vi "Start Module.vi"(6 "Show Main VI Diagram on Init (F)":bool, 8 "error in":errorcluster, 9 "Target UDP connection ref":refnum<k16>, 10 "IP:Port:Master/Slave":string, 11 "Run as Singleton? (F)":bool) -> (0 "error out":errorcluster, 1 "Wait for Event Sync?":bool, 2 "RT Interpreter Broadcast Events":T1, 3 "Module ID":i32, 4 "Module Name":string)   [LabVIEW 2021, in "RT Interpreter.lvlib"]
doc: "Launches an instance of the module Main VI. After calling this VI, you can optionally register for broadcast events from the module by wiring the broadcast events output of this VI to a <b>Register For Events</b> function. \n\nAfter the optional Register For Events function call, you should always call the <b>Synchronize Module Events.vi</b> for this module with the 'Wait for Event Sync?' output of this VI to the corresponding input of the Synchronize Module Events.vi. \n\nTo see an example of the proper wiring pattern, see the \"Run New Module: Value Change\" event frame in the API Tester VI for this module.\n\nThe <b>Validate DQMH Module</b> tool added a 'Module Name' output to this VI.\n_____\nBased on DQMH Dev Tools: Project Template 7.1.2.1547."
uses:
  RT Interpreter.lvlib
  Broadcast Events--cluster.ctl
  Did Init Argument--cluster.ctl
  Status Updated Argument--cluster.ctl
  Error Reported Argument--cluster.ctl
  Stop Argument--cluster.ctl
  Get Module Execution Status Argument--cluster.ctl
  Module Running State--enum.ctl
  <vilib>/Delacor/Delacor QMH/Libraries/Cloneable Module Admin_class/Delacor_lib_QMH_Cloneable Module Admin.lvclass
  C:/Program Files (x86)/National Instruments/LabVIEW 2021/vi.lib/Delacor/Delacor QMH/Libraries/Module Admin_class/Delacor_lib_QMH_Module Admin.lvclass
  VI Reference Management/Main VI Type--strict_vi_ref.ctl
  <vilib>/Delacor/Delacor QMH/Libraries/Cloneable Module Admin_class/Delacor_lib_QMH_Cloneable Module Admin.lvclass/Delacor_lib_QMH_Cloneable Module Admin.ctl
  <vilib>/Delacor/Delacor QMH/Libraries/Module Admin_class/Delacor_lib_QMH_Module Admin.lvclass/Delacor_lib_QMH_Module Admin.ctl
  <vilib>/Delacor/Delacor QMH/Libraries/Cloneable Module Admin_class/Delacor_lib_QMH_Set Module ID.vi
  <vilib>/Delacor/Delacor QMH/Libraries/Module Admin_class/Delacor_lib_QMH_Set External Launch.vi
  Main.vi
  Clone Registration/Clone Registration.lvlib
  VI Reference Management/VI Reference Management.lvlib
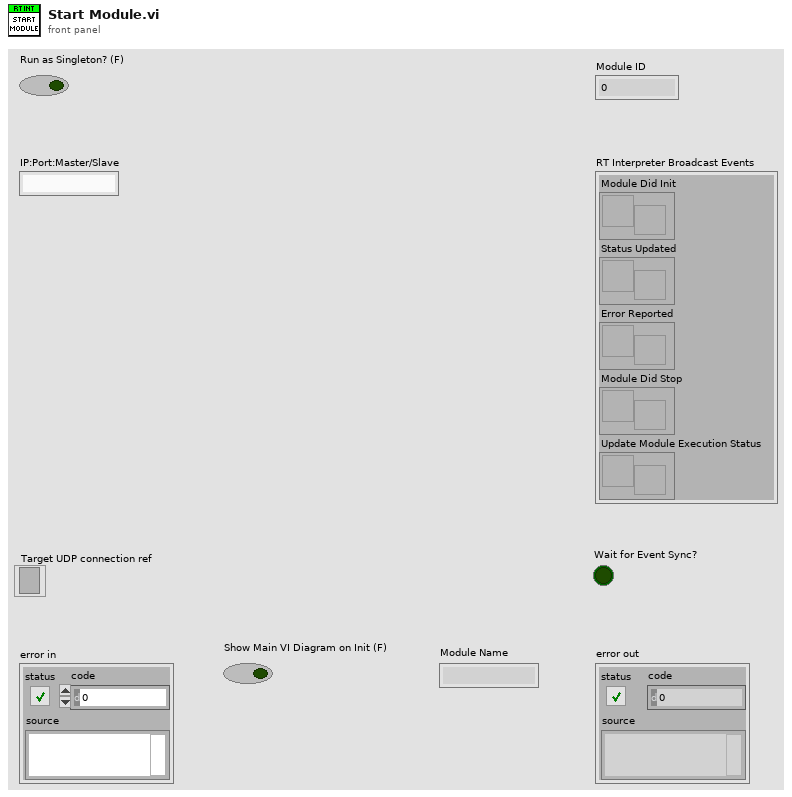
[diagram p1: front panel]
types:
  T1 = typedef "RT Interpreter.lvlib/Broadcast Events--cluster.ctl" = cluster{"Module Did Init":refnum<user-event>, "Status Updated":refnum<user-event>, "Error Reported":refnum<user-event>, "Module Did Stop":refnum<user-event>, "Update Module Execution Status":refnum<user-event>}
  T2 = typedef "RT Interpreter.lvlib/Module Running State--enum.ctl" = enum16{"Not Running", "Running as Cloneable", "Running as Singleton"}
  T3 = enum32{"Bad", "Idle", "Run top level", "Running"}
  T4 = typedef "RT Interpreter.lvlib/VI Reference Management.lvlib/Main VI Type--strict_vi_ref.ctl" = refnum<vi>
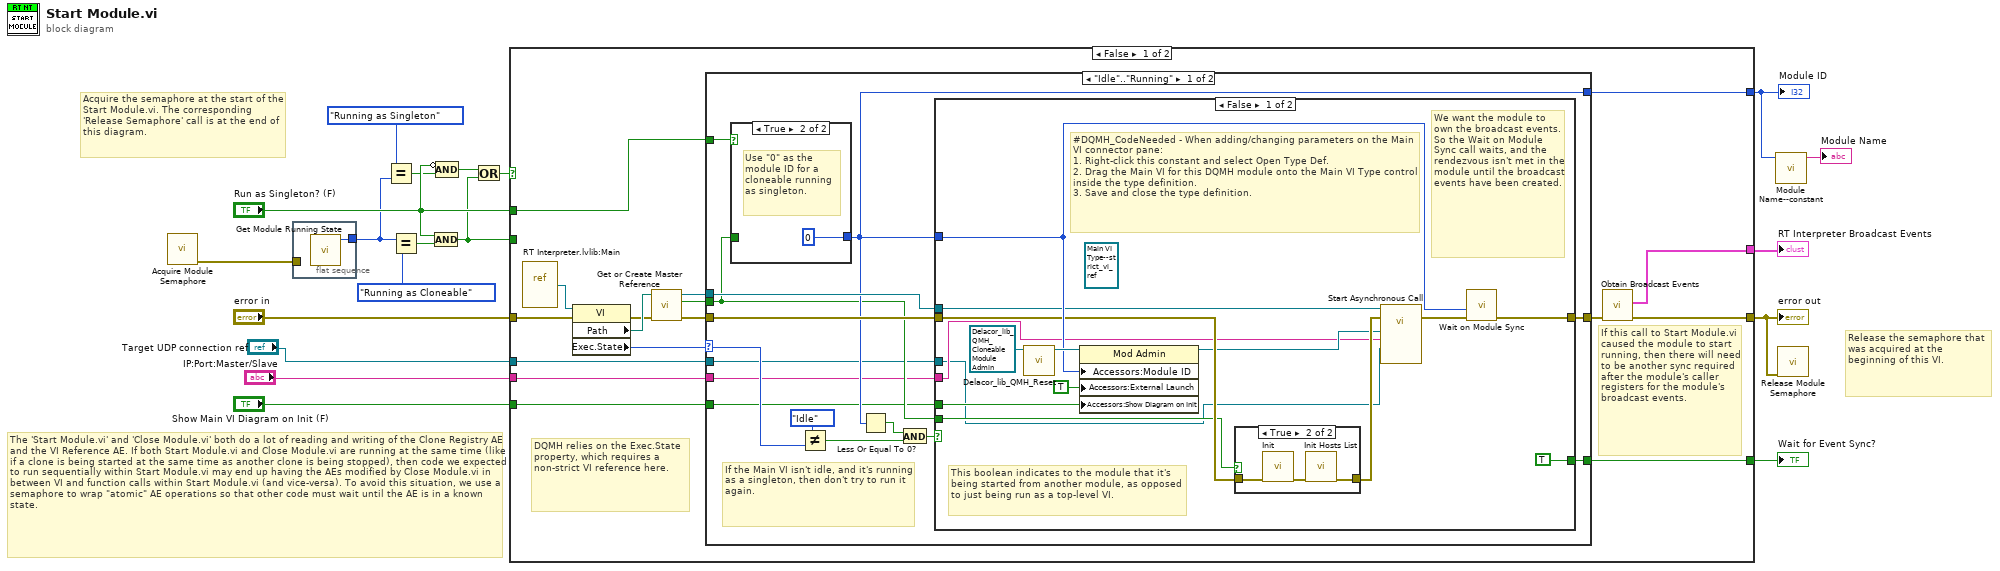
[diagram p0: block diagram]
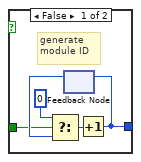
[diagram p2: hidden frame]
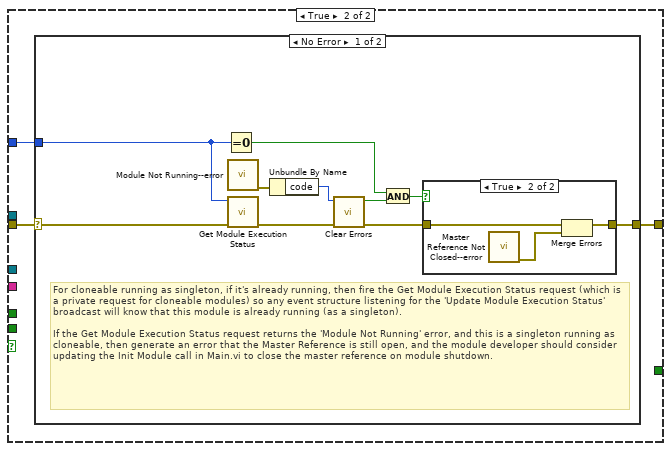
[diagram p4: hidden frame]
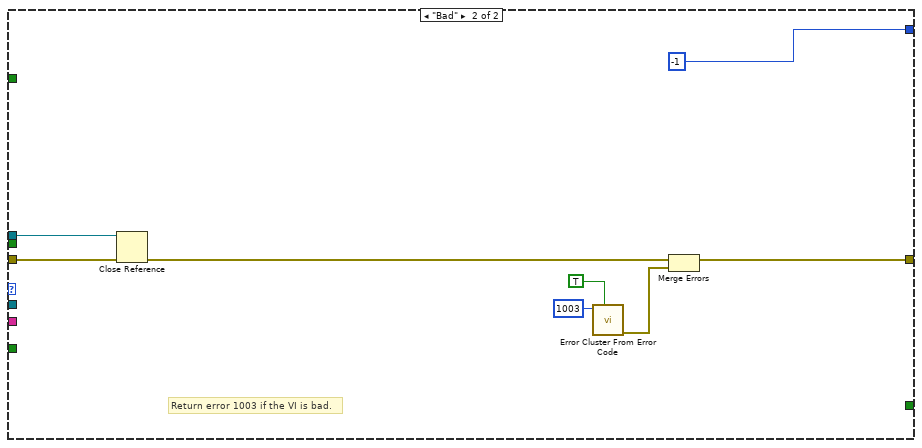
[diagram p7: hidden frame]
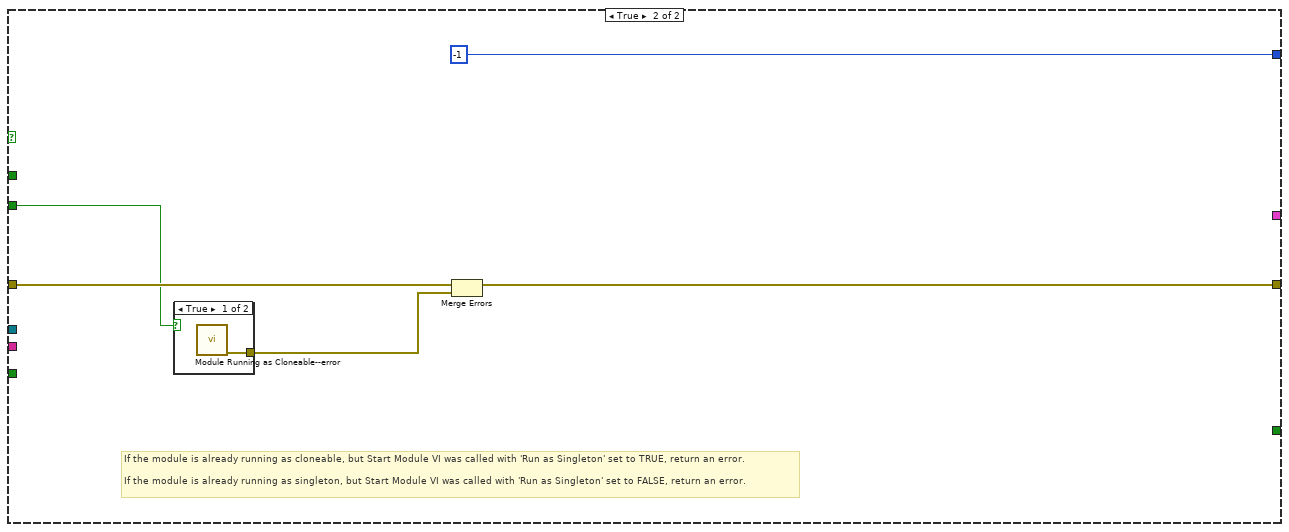
[diagram p8: hidden frame]
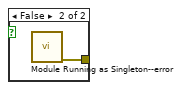
[diagram p9: hidden frame]
diagram:
  # "Release the semaphore that was acquired at the beginning of this VI."
  # "The 'Start Module.vi' and 'Close Module.vi' both do a lot of reading and writing of the Clone Registry AE and the VI Reference AE. If both Start Module.vi and Close Module.vi are running at the same time (like if a clone is being started at the same time as another clone is being stopped), then code we expected to run sequentially within Start Module.vi may end up having the AEs modified by Close Module.vi in between VI and function calls within Start Module.vi (and vice-versa). To avoid this situation, we use a semaphore to wrap \"atomic\" AE operations so that other code must wait until the AE is in a known state."
  # "Acquire the semaphore at the start of the Start Module.vi. The corresponding 'Release Semaphore' call is at the end of this diagram."
  n1 = call "Acquire Module Semaphore.vi"() -> ("error out"=w6:errorcluster)  [unwired: 11 in]
  n2 = flat-sequence {
    tunnel: [w20] -> w9
    tunnel: w6 -> [_]
    frame #0 {
      n3 = call "Get Module Running State.vi"() -> ("Module Running State"=w20:T2)  [unwired: 11 in]
    }
  }
  n4 = Equal?(x=Module_Running_State--enum."Running as Singleton", y=w9) -> (x = y?=w10:bool)
  n5 = Equal?(x=w9, y=Module_Running_State--enum."Running as Cloneable") -> (x = y?=w14:bool)
  n6 = And(x="Run as Singleton? (F)", y=w14) -> (x .and. y?=w7:bool)
  n7 = Compound Arithmetic op=AND(invert "Run as Singleton? (F)", w10) -> (w12:bool)
  n8 = Or(x=w12, y=w7) -> (x .or. y?=w13:bool)
  n9 = case shown="False" w13 {
    tunnel: "error in" -> [w37 w108]
    tunnel: [w35 w107] -> w5
    tunnel: [w34 _] -> w18
    tunnel: [w33 _] -> w17
    tunnel: [w29 -1] -> w16
    tunnel: "Run as Singleton? (F)" -> [w25 _]
    tunnel: w7 -> [_ w104]
    tunnel: "Show Main VI Diagram on Init (F)" -> [w23 _]
    tunnel: "IP:Port:Master/Slave" -> [w22 _]
    tunnel: "Target UDP connection ref" -> [w21 _]
    frame False {
      # "DQMH relies on the Exec.State property, which requires a non-strict VI reference here."
      # "If this call to Start Module.vi caused the module to start running, then there will need to be another sync required after the module's caller registers for the module's broadcast events."
      n10 = vi-ref "RT Interpreter.lvlib:Main.vi"() -> (w28:refnum<vi>)
      n11 = property class="VI"(reference=w28, error in=w37) -> (error out=w31:errorcluster, "Path"=w32:path, "Exec.State"=w26:T3)  [unwired: 1 out]
      n12 = call "Get or Create Master Reference.vi"("error in"=w31, "Main VI Path"=w32) -> ("error out"=w30:errorcluster, "New Reference Created"=w24:bool, "Master Reference"=w27:T4)  [unwired: 7 in]
      n13 = case shown="\"Idle\"..\"Running\"" w26 {
        selector: w26 -> [w48 _]
        tunnel: w30 -> [w52 w103]
        tunnel: w27 -> [w50 w102]
        tunnel: [w49 w100] -> w36
        tunnel: [w51 _] -> w33
        tunnel: [w43 -1] -> w29
        tunnel: w25 -> [w42 _]
        tunnel: w24 -> [w41 _]
        tunnel: w23 -> [w40 _]
        tunnel: w22 -> [w39 _]
        tunnel: w21 -> [w38 _]
        frame "Idle".."Running" {
          # "If the Main VI isn't idle, and it's running as a singleton, then don't try to run it again."
          n14 = case shown="True" w42 {
            tunnel: [w57 0] -> w43
            tunnel: w41 -> [w53 _]
            frame False {
              # "generate module ID"
              n15 = feedback #1() -> (w55:i32)  [unwired: 1 in]
              n16 = Select(t=0, s=w53, f=w55) -> (s? t:f=w56:i32)
              n17 = Increment(x=w56) -> (x+1=w57:i32)
              n18 = feedback-in #1(w57) -> ()
            }
            frame True {
              # "Use \"0\" as the module ID for a cloneable running as singleton."
            }
          }
          n19 = Not Equal?(x=T3."Idle", y=w48) -> (x != y?=w46:bool)
          n20 = Less Or Equal To 0?(x=w43) -> (x <= 0?=w44:bool)
          n21 = And(x=w44, y=w46) -> (x .and. y?=w45:bool)
          n22 = case shown="False" w45 {
            tunnel: w52 -> [w65 w79]
            tunnel: [TRUE _] -> w51
            tunnel: w50 -> [w64 _]
            tunnel: [w68 w78] -> w49
            tunnel: w43 -> [w69 w80]
            tunnel: w41 -> [w62 _]
            tunnel: w40 -> [w61 _]
            tunnel: w39 -> [w60 _]
            tunnel: w38 -> [w59 _]
            frame False {
              (unwired) T4 refnum ("Main VI Type")
              # "#DQMH_CodeNeeded - When adding/changing parameters on the Main VI connector pane:\n1. Right-click this constant and select Open Type Def.\n2. Drag the Main VI for this DQMH module onto the Main VI Type control inside the type definition.\n3. Save and close the type definition."
              # "We want the module to own the broadcast events. So the Wait on Module Sync call waits, and the rendezvous isn't met in the module until the broadcast events have been created."
              # "This boolean indicates to the module that it's being started from another module, as opposed to just being run as a top-level VI."
              n23 = call-dynamic "Delacor_lib_QMH_Reset.vi"("Mod Admin in"=refnum<class "Delacor_lib_QMH_Cloneable Module Admin.lvclass"> refnum) -> ("Mod Admin out"=w72:refnum<class "Delacor_lib_QMH_Cloneable Module Admin.lvclass">)  [unwired: 9 in, 1 out]
              n24 = property class="Mod Admin"(reference=w72, "Accessors:Module ID"=w69, "Accessors:External Launch"=TRUE, "Accessors:Show Diagram on Init"=w61) -> (reference out=w63:refnum<class "Delacor_lib_QMH_Cloneable Module Admin.lvclass">)  [unwired: 1 in, 1 out]
              n25 = case shown="True" w62 {
                tunnel: [w74 w75] -> w66
                tunnel: w65 -> [w74 w77]
                frame False {
                }
                frame True {
                  n26 = call "Init.vi"("error in"=w77) -> ("error out"=w76:errorcluster)  [unwired: 7 in, 3 out]
                  n27 = call "Init Hosts List.vi"("error in"=w76) -> ("error out"=w75:errorcluster)  [unwired: 10 in]
                }
              }
              n28 = call-by-ref "Start Asynchronous Call"(reference=w64, error in=w66, "Target UDP connection ref"=w59, "IP:Port:Master/Slave"=w60, "Module Admin"=w63) -> (error out=w67:errorcluster)  [unwired: 9 in, 1 out]
              n29 = call "Wait on Module Sync.vi"("error in"=w67, "Module ID"=w69) -> ("error out"=w68:errorcluster)  [unwired: 9 in]
            }
            frame True {
              n30 = case shown="No Error" w79 {
                selector: w79 -> [w90 w95]
                tunnel: w80 -> [w88 _]
                tunnel: [w81 w95] -> w78
                frame No Error {
                  # "For cloneable running as singleton, if it's already running, then fire the Get Module Execution Status request (which is a private request for cloneable modules) so any event structure listening for the 'Update Module Execution Status' broadcast will know that this module is already running (as a singleton).\n\nIf the Get Module Execution Status request returns the 'Module Not Running' error, and this is a singleton running as cloneable, then generate an error that the Master Reference is still open, and the module developer should consider updating the Init Module call in Main.vi to close the master reference on module shutdown."
                  n31 = Equal To 0?(x=w88) -> (x = 0?=w84:bool)
                  n32 = call "Module Not Running--error.vi"() -> ("error out"=w87:errorcluster)  [unwired: 11 in]
                  n33 = call "Get Module Execution Status.vi"("error in"=w90, "Module ID"=w88) -> ("error out"=w89:errorcluster)  [unwired: 9 in]
                  n34 = Unbundle By Name(w87) -> ("code"=w86:i32)
                  n35 = call <vilib>:"Clear Errors.vi"("error in (no error)"=w89, "specific error code to clear (0: all)"=w86) -> ("error out"=w83:errorcluster, "specific error cleared?"=w85:bool)  [unwired: 4 in]
                  n36 = And(x=w84, y=w85) -> (x .and. y?=w82:bool)
                  n37 = case shown="True" w82 {
                    tunnel: w83 -> [w91 w94]
                    tunnel: [w91 w92] -> w81
                    frame False {
                    }
                    frame True {
                      n38 = call "Master Reference Not Closed--error.vi"() -> ("error out"=w93:errorcluster)  [unwired: 11 in]
                      n39 = Merge Errors(w94, w93) -> (w92:errorcluster)
                    }
                  }
                }
                frame Error {
                }
              }
            }
          }
        }
        frame "Bad" {
          # "Return error 1003 if the VI is bad."
          n40 = Close Reference(reference=w102, error in (no error)=w103) -> (error out=w101:errorcluster)
          n41 = call <vilib>:"Error Cluster From Error Code.vi"("show call chain? (False)"=TRUE, "error code (0)"=1003) -> ("error out"=w98:errorcluster)  [unwired: 7 in]
          n42 = Merge Errors(w101, w98) -> (w100:errorcluster)
        }
      }
      n43 = call "Obtain Broadcast Events.vi"("error in"=w36) -> ("error out"=w35:errorcluster, "RT Interpreter Broadcast Events"=w34:T1)  [unwired: 9 in]
    }
    frame True {
      # "If the module is already running as cloneable, but Start Module VI was called with 'Run as Singleton' set to TRUE, return an error.\n\nIf the module is already running as singleton, but Start Module VI was called with 'Run as Singleton' set to FALSE, return an error."
      n44 = case shown="True" w104 {
        tunnel: [w109 w110] -> w105
        frame True {
          n45 = call "Module Running as Cloneable--error.vi"() -> ("error out"=w109:errorcluster)  [unwired: 11 in]
        }
        frame False {
          n46 = call "Module Running as Singleton--error.vi"() -> ("error out"=w110:errorcluster)  [unwired: 11 in]
        }
      }
      n47 = Merge Errors(w108, w105) -> (w107:errorcluster)
    }
  }
  "error out" <- w5
  "RT Interpreter Broadcast Events" <- w18
  "Wait for Event Sync?" <- w17
  "Module ID" <- w16
  n48 = call "Module Name--constant.vi"("Module ID"=w16) -> ("Module Name"=→"Module Name":string)  [unwired: 10 in]
  n49 = call "Release Module Semaphore.vi"("error in"=w5) -> ()  [unwired: 10 in, 1 out]
